vi "FGV Lebt der PC.vi"() -> (1 "lebt PC?":bool)   [LabVIEW 2020, in "Kommunikation mit PC.lvlib"]
uses:
  Kommunikation mit PC.lvlib
  FGV Komm Status Aktionen.ctl
  Allgemein/FGV Zustaende Aktionen.ctl
  SysLog/SysLog Interface cRIO.ctl
  Allgemein/Allgemein.lvlib
  <vilib>/nisyscfg/nisyscfg.lvlib
  SysLog/SysLog_cRIO.lvlib
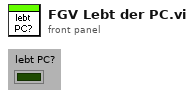
[diagram p1: front panel]
types:
  T1 = typedef "Kommunikation mit PC.lvlib/FGV Komm Status Aktionen.ctl" = enum16{"lesen", "lebt PC?"}
  T2 = typedef "Allgemein.lvlib/FGV Zustaende Aktionen.ctl" = enum16{"lesen", "Zustand PC", "Zustand cRIO", "Bildnummer", "Samplepoint", "Sysloglevel"}
  T3 = typedef "SysLog_cRIO.lvlib/SysLog Interface cRIO.ctl" = cluster{"FehlermeldungsCode":i32, "ErfolgsmeldungsCode":i32, "ParameterListenString":string, "intern":bool}
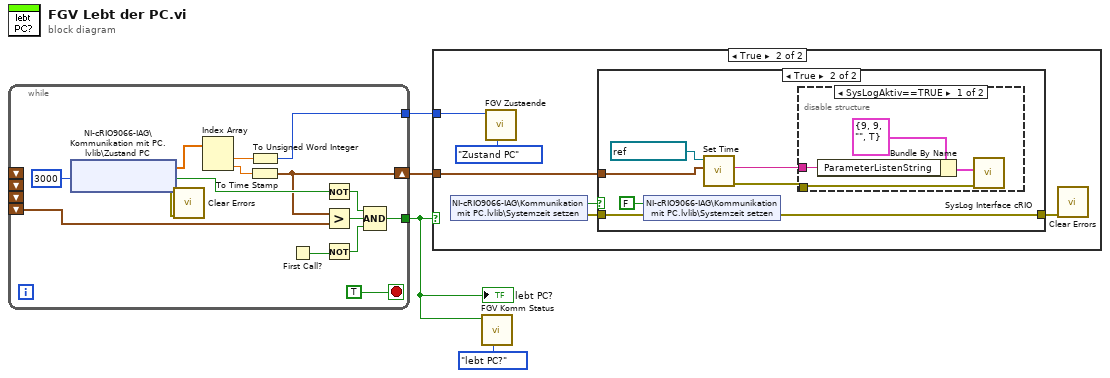
[diagram p0: block diagram]
diagram:
  n1 = while {
    shift-right: [w7] -> w3
    shift-left: _ -> [_]
    shift-left: _ -> [_]
    shift-left: _ -> [_]
    shift-left: _ -> [w15]
    tunnel: [w12] -> w1
    tunnel: [w5] -> w4
    stop <- TRUE stop-if-true
    n2 = shared-variable "NI-cRIO9066-IAG\\Kommunikation mit PC.lvlib\\Zustand PC"(3000 ("Timeout in ms(0)")) -> (w8:dbl[], error out=w6:errorcluster, w14:bool)  [unwired: 1 out]
    n3 = call <vilib>:"Clear Errors.vi"("error in (no error)"=w6) -> ()  [unwired: 5 in, 2 out]
    n4 = Index Array(array=w8) -> (element #1=w9:dbl, element #2=w10:dbl)  [unwired: 2 in]
    n5 = To Unsigned Word Integer(number=w9) -> (unsigned 16bit integer=w5:u16)
    n6 = To Time Stamp(1:w10) -> (0:w7:timestamp)
    n7 = First Call?() -> (First Call?: T/F=w18:bool)
    n8 = Not(x=w14) -> (.not. x?=w13:bool)
    n9 = Greater?(x=w7, y=w15) -> (0:w16:bool)
    n10 = Not(x=w18) -> (.not. x?=w17:bool)
    n11 = Compound Arithmetic op=AND(w13, w16, w17) -> (w12:bool)
  }
  "lebt PC?" <- w1
  n12 = case shown="True" w1 {
    tunnel: w4 -> [_ w21]
    tunnel: w3 -> [_ w24]
    frame False {
    }
    frame True {
      n13 = shared-variable "NI-cRIO9066-IAG\\Kommunikation mit PC.lvlib\\Systemzeit setzen"() -> (w25:bool, error out=w23:errorcluster)  [unwired: 1 in]
      n14 = call "FGV Zustaende.vi"("Aktionen"=FGV_Zustaende_Aktionen."Zustand PC", "Zustand PC"=w21) -> ()  [unwired: 5 in, 5 out]
      n15 = case shown="True" w25 {
        tunnel: w24 -> [_ w29]
        tunnel: w23 -> [w26 w32]
        tunnel: [w26 w31] -> w20
        frame False {
        }
        frame True {
          n16 = shared-variable "NI-cRIO9066-IAG\\Kommunikation mit PC.lvlib\\Systemzeit setzen"(FALSE ("Systemzeit setzen"), error in=w32) -> (error out=w31:errorcluster)
          n17 = call <vilib>:"Set Time.vi"("Time"=w29, "Session in (localhost)"=refnum<k21> "localhost" ("session in (localhost)")) -> ("error out"=w28:errorcluster, "Detailed Result"=w27:string)  [unwired: 6 in, 2 out]
          n18 = disable-structure shown="SysLogAktiv==TRUE" {
            disable-tunnel: w28 -> [w37 _]
            disable-tunnel: w27 -> [w34 _]
            frame condition #0 (active) {
              n19 = Bundle By Name(cluster=T3 {"FehlermeldungsCode"=9, "ErfolgsmeldungsCode"=9, "ParameterListenString"="", "intern"=TRUE} ("Cluster (in)"), "ParameterListenString"=w34) -> (w35:T3)
              n20 = call "SysLog Interface cRIO.vi"("Fehler (in)"=w37, "Cluster (in)"=w35) -> ()  [unwired: 9 in, 1 out]
            }
            frame condition #1 {
            }
          }
        }
      }
      n21 = call <vilib>:"Clear Errors.vi"("error in (no error)"=w20) -> ()  [unwired: 5 in, 2 out]
    }
  }
  n22 = call "FGV Komm Status.vi"("Aktionen"=FGV_Komm_Status_Aktionen."lebt PC?", "lebt PC?"=w1) -> ()  [unwired: 9 in, 1 out]
